vi "Round to Increment.vi"(1 "Input":dbl) -> (0 "Output":dbl)   [LabVIEW 2014]
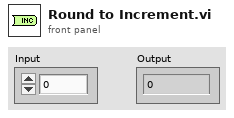
[diagram p1: front panel]
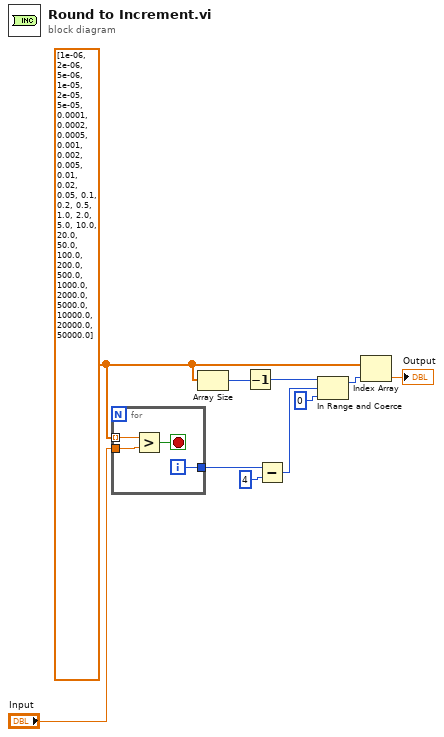
[diagram p0: block diagram]
diagram:
  w8 = dbl[] [1e-06, 2e-06, 5e-06, 1e-05, 2e-05, 5e-05, 0.0001, 0.0002, 0.0005, 0.001, 0.002, 0.005, 0.01, 0.02, 0.05, 0.1, 0.2, 0.5, 1.0, 2.0, 5.0, 10.0, 20.0, 50.0, 100.0, 200.0, 500.0, 1000.0, 2000.0, 5000.0, 10000.0, 20000.0, 50000.0]
  n1 = for {
    tunnel: w8 -> [w14] mode=indexing
    tunnel: "Input" -> [w13]
    tunnel: [w11] -> w2
    i -> [w11]
    stop <- w12 stop-if-true
    n2 = Greater?(x=w14, y=w13) -> (0:w12:bool)
  }
  n3 = Array Size(array=w8) -> (size(s)=w9:i32)
  n4 = Decrement(x=w9) -> (x-1=w10:i32)
  n5 = Subtract(x=w2, y=4 ("x")) -> (x-y=w5:i32)
  n6 = In Range and Coerce(upper limit=w10, x=w5, lower limit=0) -> (coerced(x)=w7:i32)  [unwired: 1 out]
  n7 = Index Array(array=w8, index=w7) -> (element=→"Output":dbl)
